vi "SetImgToImgCtrl.vi"(7 "type":T1(ring), 10 "img file path":path, 11 "ref img in":refnum<vi>) -> (3 "ref img out":refnum<vi>)   [LabVIEW 2018, in "Library-Ctrl.lvlib"]
uses:
  Library-Ctrl.lvlib
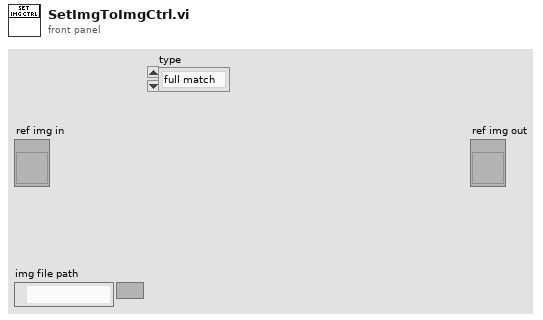
[diagram p1: front panel]
types:
  T1 = enum16{"full match", "height match", "width match"}
  T2 = typedef "imagedata.ctl" = cluster{"image type":i32, "image depth":i32, "image":u8[], "mask":u8[], "colors":u32[], "Rectangle":cluster{"left":i16, "top":i16, "right":i16, "bottom":i16}}
  T3 = typedef "LVBoundsTypeDef.ctl" = cluster{"Width":u32, "Height":u32}
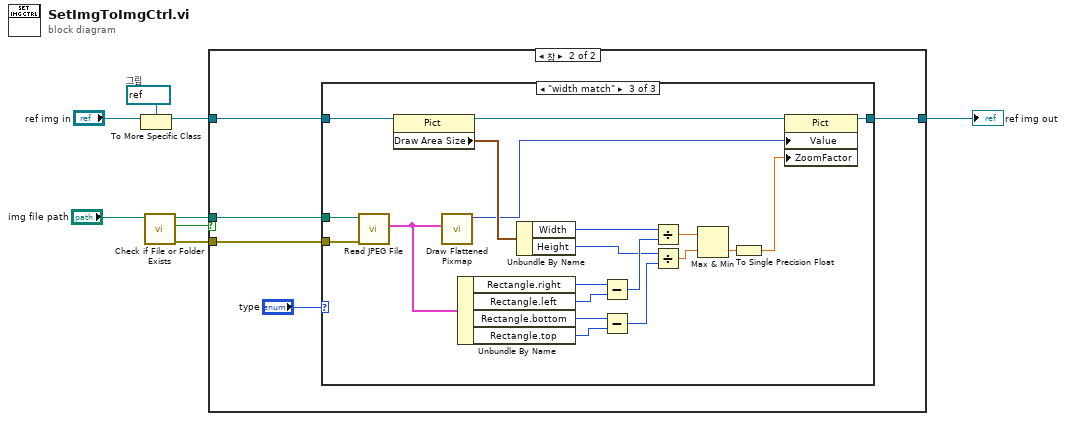
[diagram p0: block diagram]
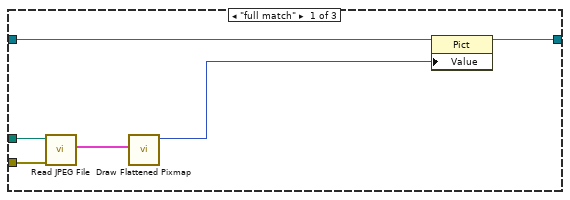
[diagram p3: hidden frame]
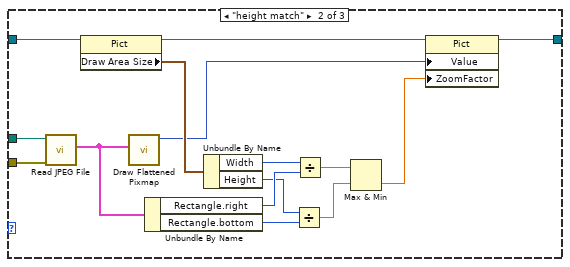
[diagram p4: hidden frame]
diagram:
  w3 = refnum<vi> refnum  # 그림
  n1 = To More Specific Class(target class=w3, reference="ref img in") -> (specific class reference=w2:refnum<vi>)  [unwired: 1 in, 1 out]
  n2 = call <vilib>:"Check if File or Folder Exists.vi"("path"="img file path") -> ("error out"=w5:errorcluster, "file or folder exists?"=w7:bool, "dup path"=w6:path)  [unwired: 8 in]
  n3 = case shown="참" w7 {
    tunnel: w6 -> [_ w14]
    tunnel: w5 -> [_ w13]
    tunnel: w2 -> [w9 w12]
    tunnel: [w9 w11] -> w1
    frame False {
    }
    frame True {
      n4 = case shown="\"width match\"" "type" {
        tunnel: w14 -> [w20 w35 w55]
        tunnel: w13 -> [w19 w34 w54]
        tunnel: w12 -> [w15 w32 w52]
        tunnel: [w16 w21 w48] -> w11
        frame "full match" {
          n5 = call <vilib>:"Read JPEG File.vi"("error in (no error)"=w19, "path to JPEG file"=w20) -> ("image data"=w18:T2)  [unwired: 7 in, 2 out]
          n6 = call <vilib>:"Draw Flattened Pixmap.vi"("image data"=w18) -> ("new picture"=w17:picture)  [unwired: 8 in]
          n7 = property class="Pict"(reference=w15, "Value"=w17) -> (reference out=w16:refnum<vi>)  [unwired: 1 in, 1 out]
        }
        frame "height match" {
          n8 = call <vilib>:"Read JPEG File.vi"("error in (no error)"=w34, "path to JPEG file"=w35) -> ("image data"=w33:T2)  [unwired: 7 in, 2 out]
          n9 = property class="Pict"(reference=w32) -> (reference out=w31:refnum<vi>, "Draw Area Size"=w30:T3)  [unwired: 1 in, 1 out]
          n10 = call <vilib>:"Draw Flattened Pixmap.vi"("image data"=w33) -> ("new picture"=w29:picture)  [unwired: 8 in]
          n11 = Unbundle By Name(w33) -> ("Rectangle.right"=w27:i16, "Rectangle.bottom"=w26:i16)
          n12 = Unbundle By Name(w30) -> ("Width"=w28:u32, "Height"=w25:u32)
          n13 = Divide(x=w25, y=w26) -> (x/y=w23:dbl)
          n14 = Divide(x=w28, y=w27) -> (x/y=w24:dbl)
          n15 = Max & Min(x=w24, y=w23) -> (min(x,y)=w22:dbl)  [unwired: 1 out]
          n16 = property class="Pict"(reference=w31, "Value"=w29, "ZoomFactor"=w22) -> (reference out=w21:refnum<vi>)  [unwired: 1 in, 1 out]
        }
        frame "width match" {
          n17 = call <vilib>:"Read JPEG File.vi"("error in (no error)"=w54, "path to JPEG file"=w55) -> ("image data"=w53:T2)  [unwired: 7 in, 2 out]
          n18 = property class="Pict"(reference=w52) -> (reference out=w51:refnum<vi>, "Draw Area Size"=w50:T3)  [unwired: 1 in, 1 out]
          n19 = call <vilib>:"Draw Flattened Pixmap.vi"("image data"=w53) -> ("new picture"=w49:picture)  [unwired: 8 in]
          n20 = Unbundle By Name(w53) -> ("Rectangle.right"=w47:i16, "Rectangle.left"=w46:i16, "Rectangle.bottom"=w45:i16, "Rectangle.top"=w44:i16)
          n21 = Unbundle By Name(w50) -> ("Width"=w43:u32, "Height"=w41:u32)
          n22 = Subtract(x=w47, y=w46) -> (x-y=w42:i16)
          n23 = Subtract(x=w45, y=w44) -> (x-y=w40:i16)
          n24 = Divide(x=w43, y=w42) -> (x/y=w39:dbl)
          n25 = Divide(x=w41, y=w40) -> (x/y=w38:dbl)
          n26 = Max & Min(x=w39, y=w38) -> (min(x,y)=w37:dbl)  [unwired: 1 out]
          n27 = To Single Precision Float(number=w37) -> (single precision float=w36:sgl)
          n28 = property class="Pict"(reference=w51, "Value"=w49, "ZoomFactor"=w36) -> (reference out=w48:refnum<vi>)  [unwired: 1 in, 1 out]
        }
      }
    }
  }
  "ref img out" <- w1
